vi "find_incidence_angles.vi"(11 "Light positions":sgl[][](array[numeric])) -> (3 "Incidence angles":dbl[][](array[numeric]))   [LabVIEW 2013]
uses:
  <vilib>/Analysis/baseanly.llb/Real Dot Product.vi
  initialization/micron_globals.vi
  utilities/labview/norm_vec.vi
  <vilib>/Analysis/NI_AALBase.lvlib
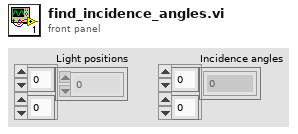
[diagram p1: front panel]
types:
  T1 = typedef "configuration.ctl" = cluster{"Calibration data":T2, "Block size":i32, "Tasks":cluster{"Analog Input":refnum<k21>, "Counters":refnum<k21>[], "Digital out":refnum<k21>}, "Light enables":bool[]}
  T2 = typedef "asap_calibration.ctl" = cluster{"T1":T3, "K1":T3, "T2":T3, "K2":T3, "Sensor LUT":sgl[][][][]}
  T3 = typedef "NI_Matrix.lvlib/RealMatrix.ctl" = dbl[][]
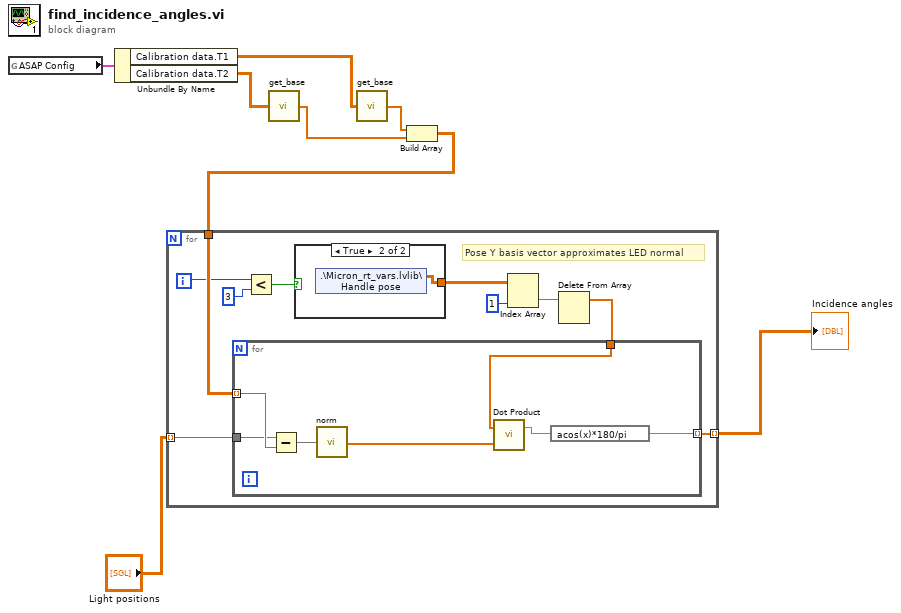
[diagram p0: block diagram]
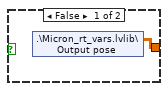
[diagram p2: hidden frame]
diagram:
  n1 = global read "micron_globals.vi" "ASAP Config"() -> (w5:T1)
  n2 = Unbundle By Name(w5) -> ("Calibration data.T1"=w4:T3, "Calibration data.T2"=w3:T3)
  n3 = call "get_base.vi"("T"=w3) -> ("Array"=w7:dbl[])
  n4 = call "get_base.vi"("T"=w4) -> ("Array"=w6:dbl[])
  n5 = Build Array(w6, w7) -> (w8:dbl[][])
  n6 = for {
    tunnel: "Light positions" -> [w17] mode=indexing
    tunnel: w8 -> [w18]
    tunnel: [w16] -> w1 mode=indexing
    i -> [w15]
    # "Pose Y basis vector approximates LED normal"
    n7 = Less?(x=w15, y=3) -> (x < y?=w13:bool)
    n8 = case shown="True" w13 {
      tunnel: [w19 w20] -> w10
      frame False {
        n9 = shared-variable ".\\Micron_rt_vars.lvlib\\Output pose"() -> (w19:sgl[][])  [unwired: 1 in, 1 out]
      }
      frame True {
        n10 = shared-variable ".\\Micron_rt_vars.lvlib\\Handle pose"() -> (w20:sgl[][])  [unwired: 1 in, 1 out]
      }
    }
    n11 = Index Array(array=w10, index (col)=1 ("disabled index (col)")) -> (element=w12:sgl[])  [unwired: 1 in]
    n12 = Delete From Array(array=w12) -> (array with subset deleted=w9:sgl[])  [unwired: 2 in, 1 out]
    n13 = for {
      tunnel: w18 -> [w27] mode=indexing
      tunnel: w17 -> [w26]
      tunnel: w9 -> [w24]
      tunnel: [w21] -> w16 mode=indexing
      n14 = Subtract(x=w26, y=w27) -> (x-y=w25:dbl[])
      n15 = call-poly "norm.vi"("vector"=w25) -> ("normalized vector"=w23:dbl[])  [unwired: 3 in, 1 out]
      n16 = call-poly <vilib>:"Dot Product.vi"("Y Vector"=w23, "X Vector"=w24) -> ("X * Y"=w22:dbl)  [unwired: 1 out]
      n17 = expression code="acos(x)*180/pi"(w22) -> (w21:dbl)
    }
  }
  "Incidence angles" <- w1
